vi "Begin.vi"(8 "error in":errorcluster) -> (0 "error out":errorcluster)   [LabVIEW 2015]
doc: "Called before other user functions, this VI is expected to open initial I/O refnums, load in file data, and do all program initialization. Notice that the <B>error out</B> terminal is simply used for data flow. Wiring it to other structures or subVIs ensures that this VI runs first."
uses:
  <vilib>/Rock Robotics/WPI/DriverStation/WPI_DriverStationRobotMode2.ctl
  <vilib>/Rock Robotics/WPI/Joystick/WPI_JoystickDeviceEnum.ctl
  <vilib>/Rock Robotics/WPI/Solenoid/WPI_SolenoidChannel.ctl
  <vilib>/Rock Robotics/SystemInterfaces/DIO/FPGA_DIOPWMChannel.ctl
  <vilib>/Rock Robotics/WPI/SafetyOutput/WPI_SafetyOutputConfigMenu.ctl
  Robot Global Data.vi
  <vilib>/Rock Robotics/Network Tables/NT Write String Array.vi
  <vilib>/Rock Robotics/WPI/Solenoid/WPI_SolenoidOpenSingle.vi
  <vilib>/Rock Robotics/WPI/MotorControl/WPI_MotorControlOpen Talon.vi
  <vilib>/Rock Robotics/WPI/MotorControl/WPI_MotorControlOpenCANTalonSRX.vi
  <vilib>/Rock Robotics/WPI/RobotDrive/WPI_RobotDriveOpen4MotorWithCANTalonSRX.vi
  <vilib>/Rock Robotics/WPI/Counter/WPI_CounterDigitalInputToDigitalSource.vi
  <vilib>/Rock Robotics/SystemInterfaces/DIO/FPGA_DIOChannel.ctl
  <vilib>/Rock Robotics/WPI/MotorControl/WPI_MotorControlOpen Victor.vi
  <vilib>/Rock Robotics/WPI/Gyro/WPI_GyroAnalogOpen.vi
  <vilib>/Rock Robotics/SystemInterfaces/AI/FPGA_AIGyroChannel.ctl
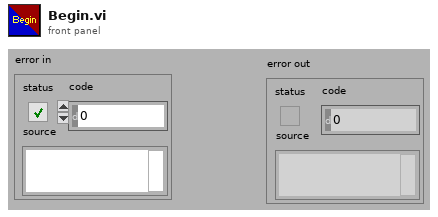
[diagram p1: front panel]
types:
  T1 = typedef "WPI_SafetyOutputConfigMenu.ctl" = enum16{"Enable", "Disable"}
  T2 = typedef "WPI_SolenoidChannel.ctl" = enum8{"Solenoid 0", "Solenoid 1", "Solenoid 2", "Solenoid 3", "Solenoid 4", "Solenoid 5", "Solenoid 6", "Solenoid 7", "Invalid"}
  T3 = typedef "FPGA_DIOPWMChannel.ctl" = enum8{"PWM 0", "PWM 1", "PWM 2", "PWM 3", "PWM 4", "PWM 5", "PWM 6", "PWM 7", "PWM 8", "PWM 9", "PWM MXP 0", "PWM MXP 1", "PWM MXP 2", "PWM MXP 3", "PWM MXP 4", "PWM MXP 5", "PWM MXP 6", "PWM MXP 7", "PWM MXP 8", "PWM MXP 9", "Invalid"}
  T4 = typedef "WPI_JoystickDeviceEnum.ctl" = enum16{"USB 0", "USB 1", "USB 2", "USB 3", "USB 4", "USB 5"}
  T5 = typedef "WPI_DriverStationRobotMode2.ctl" = enum16{"Autonomous Disabled", "Autonomous Enabled", "Teleop Disabled", "Teleop Enabled", "Disconnected", "Finish", "Test Disabled", "Test Enabled", "Emergency Stopped"}
  T6 = typedef "FPGA_DIOChannel.ctl" = enum8{"DIO 0", "DIO 1", "DIO 2", "DIO 3", "DIO 4", "DIO 5", "DIO 6", "DIO 7", "DIO 8", "DIO 9", "DIO MXP 0", "DIO MXP 1", "DIO MXP 2", "DIO MXP 3", "DIO MXP 4", "DIO MXP 5", "DIO MXP 6", "DIO MXP 7", "DIO MXP 8", "DIO MXP 9", "DIO MXP 10", "DIO MXP 11", "DIO MXP 12", "DIO MXP 13", "DIO MXP 14", "DIO MXP 15", "Invalid"}
  T7 = typedef "WPI_DigitalInputDevRef.ctl" = cluster{"DevStatus":errorcluster, "DIO Channel":T6}
  T8 = typedef "FPGA_CounterEncoderSourceConvertionLVSourceType.ctl" = cluster{"DevStatus":errorcluster, "AnalogTriggerMode?":bool, "DigitalMode":cluster{"DIO Channel":T9}, "AnalogTriggerMode":cluster{"AnalogTriggerIndex":T10, "OutputType":T11}}
  T9 = typedef "FPGA_DIODigitalSourceChannel.ctl" = enum8{"DIO 0", "DIO 1", "DIO 2", "DIO 3", "DIO 4", "DIO 5", "DIO 6", "DIO 7", "DIO 8", "DIO 9", "DIO MXP 0", "DIO MXP 1", "DIO MXP 2", "DIO MXP 3", "DIO MXP 4", "DIO MXP 5", "DIO MXP 6", "DIO MXP 7", "DIO MXP 8", "DIO MXP 9", "DIO MXP 10", "DIO MXP 11", "DIO MXP 12", "DIO MXP 13", "DIO MXP 14", "DIO MXP 15", "Disabled"}
  T10 = typedef "FPGA_AnalogTriggerIndex.ctl" = enum8{"Trig 0", "Trig 1", "Trig 2", "Trig 3", "Trig 4", "Trig 5", "Trig 6", "Trig 7", "Invalid"}
  T11 = typedef "FPGA_AnalogTriggerOutType.ctl" = enum16{"InWindow", "TriggerState", "Rising", "Falling"}
  T12 = typedef "WPI_EncoderDevRef.ctl" = cluster{"DevStatus":errorcluster, "EncoderIndex":T13, "CounterIndex":T14, "DistancePerCount":dbl, "Decoding Type":T15}
  T13 = typedef "FPGA_EncoderIdx.ctl" = enum8{"Enc 0", "Enc 1", "Enc 2", "Enc 3", "Enc 4", "Enc 5", "Enc 6", "Enc 7", "Invalid"}
  T14 = typedef "FPGA_CounterCtrSystemIndex.ctl" = enum8{"Ctr 0", "Ctr 1", "Ctr 2", "Ctr 3", "Ctr 4", "Ctr 5", "Ctr 6", "Ctr 7", "Invalid"}
  T15 = typedef "WPI_EncoderType.ctl" = enum16{"1x", "2x", "4x"}
  T16 = typedef "WPI_JoystickDevRef.ctl" = cluster{"Device":T4}
  T17 = typedef "WPI_SolenoidDevRef.ctl" = cluster{"DevStatus":errorcluster, "Pneumatics Control Module":u8, "Forward Solenoid Channel":T2, "Reverse Solenoid Channel":T2}
  T18 = typedef "WPI_MotorControlDeviceRef.ctl" = cluster{"DeviceStatus":errorcluster, "Type":T19, "PWM":cluster{"PWM Channel":T3, "DeadBand":T20}, "CAN":cluster{"Device Number":u8, "Control Mode":T21, "Semaphore":T22, "Max Vout":dbl, "TalonSRX Control Mode":T23}, "Invert":bool}
  T19 = typedef "WPI_MotorControlType.ctl" = enum16{"PWM", "CAN", "CANTalonSRX"}
  T20 = typedef "WPI_PWMDeadband.ctl" = cluster{"Name":string, "maxPositivePwm":i32, "minPositivePwm":i32, "centerPwm":i32, "maxNegativePwm":i32, "minNegativePwm":i32, "angularRange":u16}
  T21 = typedef "WPI_CANJaguar_ControlMode.ctl" = enum8{"Percent VBus", "Current", "Speed", "Position", "Voltage"}
  T22 = typedef "Semaphore RefNum" = refnum<k1>
  T23 = typedef "WPI_CANTalonSRX_APIControlMode.ctl" = enum8{"Percent VBus", "Speed", "Position", "Slave", "Unchanged / Invalid", "Voltage Compensation", "Current", "Motion Profile"}
  T24 = typedef "FPGA_AIGyroChannel.ctl" = enum8{"AI 0", "AI 1", "Invalid"}
  T25 = typedef "WPI_GyroDevRef.ctl" = cluster{"DevStatus":errorcluster, "Analog Channel":T26, "Offset":dbl, "Gain (VoltsPerDegree/Second)":dbl, "Gyro Type":enum16{"Analog", "XRS450"}, "Handle":i32, "SPI Bus":T27, "Device Found":bool, "Sample Rate":dbl, "Calibrate On Open":bool}
  T26 = typedef "FPGA_AIChannel.ctl" = enum8{"AI 0", "AI 1", "AI 2", "AI 3", "AI MXP 0", "AI MXP 1", "AI MXP 2", "AI MXP 3", "Invalid"}
  T27 = typedef "spi_bus.ctl" = enum16{"SPI On-Board, CS0", "SPI On-Board, CS1", "SPI On-Board, CS2", "SPI On-Board, CS3", "SPI MXP", "Invalid"}
  T28 = typedef "WPI_RobotDriveDevRef.ctl" = cluster{"DevStatus":errorcluster, "Motors[]":T18[], "Square Inputs":bool, "Max Output":dbl}
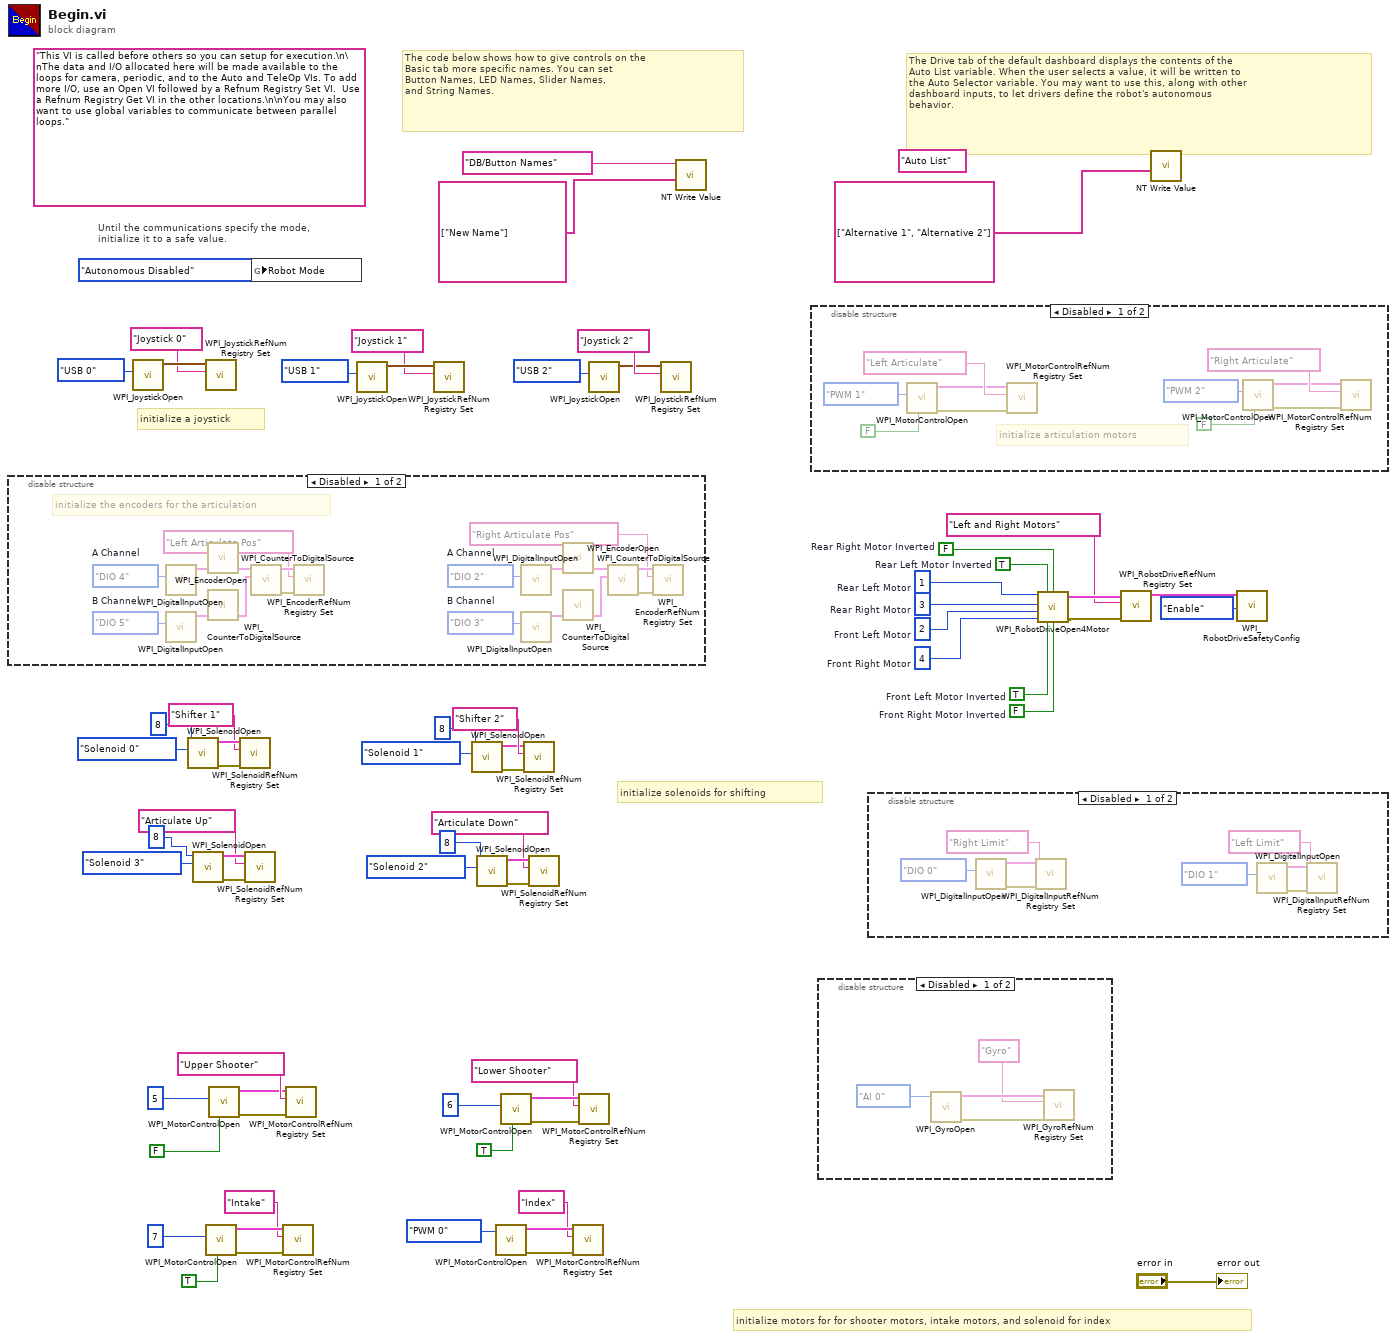
[diagram p0: block diagram]
diagram:
  w13 = u8 4  # Front Right Motor
  w12 = u8 3  # Rear Right Motor
  w11 = u8 2  # Front Left Motor
  w10 = u8 1  # Rear Left Motor
  w9 = TRUE  # Rear Left Motor Inverted
  w8 = FALSE  # Rear Right Motor Inverted
  w7 = FALSE  # Front Right Motor Inverted
  w6 = TRUE  # Front Left Motor Inverted
  (unwired) "This VI is called before others so you can setup for execution.\n\nThe data and I/O allocated here will be made available to the loops for camera, periodic, and to the Auto and TeleOp VIs. To add more I/O, use an Open VI followed by a Refnum Registry Set VI.  Use a Refnum Registry Get VI in the other locations.\n\nYou may also want to use global variables to communicate between parallel loops."
  # "initialize solenoids for shifting"
  # "initialize a joystick"
  # "initialize motors for for shooter motors, intake motors, and solenoid for index"
  # "The Drive tab of the default dashboard displays the contents of the\nAuto List variable. When the user selects a value, it will be written to\nthe Auto Selector variable. You may want to use this, along with other\ndashboard inputs, to let drivers define the robot's autonomous\nbehavior."
  # "The code below shows how to give controls on the\nBasic tab more specific names. You can set\nButton Names, LED Names, Slider Names,\nand String Names."
  # "Until the communications specify the mode,\ninitialize it to a safe value."
  n1 = disable-structure shown="Disabled" {
    frame Disabled {
      w69 = FPGA_DIOChannel."DIO 5"  # B Channel
      w70 = FPGA_DIOChannel."DIO 4"  # A Channel
      w85 = FPGA_DIOChannel."DIO 3"  # B Channel
      w84 = FPGA_DIOChannel."DIO 2"  # A Channel
      # "initialize the encoders for the articulation"
      n2 = call <vilib>:"WPI_DigitalInputOpen.vi"("DIO Channel"=w70) -> ("DigitalInputDevRef"=w73:T7)  [unwired: 1 in, 9 out]
      n3 = call <vilib>:"WPI_DigitalInputOpen.vi"("DIO Channel"=w69) -> ("DigitalInputDevRef"=w72:T7)  [unwired: 1 in, 9 out]
      n4 = call-poly <vilib>:"WPI_CounterToDigitalSource.vi"("DigitalInputDevRef"=w73) -> ("Digital Source"=w74:T8)  [unwired: 6 out]
      n5 = call-poly <vilib>:"WPI_CounterToDigitalSource.vi"("DigitalInputDevRef"=w72) -> ("Digital Source"=w71:T8)  [unwired: 6 out]
      n6 = call <vilib>:"WPI_EncoderOpen.vi"("BSource"=w71, "ASource"=w74) -> ("error out"=w75:errorcluster, "EncoderDevRef"=w76:T12)  [unwired: 6 in, 2 out]
      n7 = call <vilib>:"WPI_EncoderRefNum Registry Set.vi"("error in (no error)"=w75, "refnum name"="Left Articulate Pos", "EncoderDevRef"=w76) -> ()  [unwired: 7 in, 2 out]
      n8 = call <vilib>:"WPI_DigitalInputOpen.vi"("DIO Channel"=w84) -> ("DigitalInputDevRef"=w81:T7)  [unwired: 1 in, 9 out]
      n9 = call <vilib>:"WPI_DigitalInputOpen.vi"("DIO Channel"=w85) -> ("DigitalInputDevRef"=w82:T7)  [unwired: 1 in, 9 out]
      n10 = call-poly <vilib>:"WPI_CounterToDigitalSource.vi"("DigitalInputDevRef"=w81) -> ("Digital Source"=w80:T8)  [unwired: 6 out]
      n11 = call-poly <vilib>:"WPI_CounterToDigitalSource.vi"("DigitalInputDevRef"=w82) -> ("Digital Source"=w83:T8)  [unwired: 6 out]
      n12 = call <vilib>:"WPI_EncoderOpen.vi"("BSource"=w83, "ASource"=w80) -> ("error out"=w79:errorcluster, "EncoderDevRef"=w78:T12)  [unwired: 6 in, 2 out]
      n13 = call <vilib>:"WPI_EncoderRefNum Registry Set.vi"("error in (no error)"=w79, "refnum name"="Right Articulate Pos", "EncoderDevRef"=w78) -> ()  [unwired: 7 in, 2 out]
    }
    frame Enabled {
    }
  }
  n14 = call <vilib>:"WPI_JoystickOpen.vi"("JoystickDevice"=WPI_JoystickDeviceEnum."USB 0") -> ("JoystickDevRef"=w60:T16)  [unwired: 10 in]
  n15 = call-poly <vilib>:"WPI_SolenoidOpen.vi"("Solenoid Channel"=WPI_SolenoidChannel."Solenoid 0", "Pneumatics Control Module (0)"=u8 8) -> ("error out"=w52:errorcluster, "SolenoidDevRef"=w51:T17)  [unwired: 8 in]
  n16 = call-poly <vilib>:"WPI_SolenoidOpen.vi"("Solenoid Channel"=WPI_SolenoidChannel."Solenoid 3", "Pneumatics Control Module (0)"=u8 8) -> ("error out"=w32:errorcluster, "SolenoidDevRef"=w33:T17)  [unwired: 8 in]
  n17 = call <vilib>:"WPI_JoystickRefNum Registry Set.vi"("refnum name"="Joystick 0", "JoystickDevRef"=w60) -> ()  [unwired: 8 in, 2 out]
  n18 = call-poly <vilib>:"WPI_MotorControlOpen.vi"("Invert"=TRUE, "Device Number"=u8 7) -> ("error out"=w18:errorcluster, "MotorControlDeviceRef"=w17:T18)  [unwired: 8 in]
  n19 = call-poly <vilib>:"WPI_MotorControlOpen.vi"("Invert"=FALSE, "Device Number"=u8 5) -> ("error out"=w26:errorcluster, "MotorControlDeviceRef"=w27:T18)  [unwired: 8 in]
  n20 = call <vilib>:"WPI_SolenoidRefNum Registry Set.vi"("error in (no error)"=w52, "refnum name"="Shifter 1", "SolenoidDevRef"=w51) -> ()  [unwired: 7 in, 2 out]
  n21 = call <vilib>:"WPI_SolenoidRefNum Registry Set.vi"("error in (no error)"=w32, "refnum name"="Articulate Up", "SolenoidDevRef"=w33) -> ()  [unwired: 7 in, 2 out]
  n22 = global write "Robot Global Data.vi" "Robot Mode"(WPI_DriverStationRobotMode2."Autonomous Disabled" ("Robot Mode")) -> ()
  n23 = call <vilib>:"WPI_MotorControlRefNum Registry Set.vi"("error in (no error)"=w18, "refnum name"="Intake", "MotorControlDevRef"=w17) -> ()  [unwired: 7 in, 2 out]
  n24 = call <vilib>:"WPI_MotorControlRefNum Registry Set.vi"("error in (no error)"=w26, "refnum name"="Upper Shooter", "MotorControlDevRef"=w27) -> ()  [unwired: 7 in, 2 out]
  n25 = call <vilib>:"WPI_JoystickOpen.vi"("JoystickDevice"=WPI_JoystickDeviceEnum."USB 1") -> ("JoystickDevRef"=w57:T16)  [unwired: 10 in]
  n26 = call <vilib>:"WPI_JoystickRefNum Registry Set.vi"("refnum name"="Joystick 1", "JoystickDevRef"=w57) -> ()  [unwired: 8 in, 2 out]
  n27 = call-poly <vilib>:"WPI_SolenoidOpen.vi"("Solenoid Channel"=WPI_SolenoidChannel."Solenoid 1", "Pneumatics Control Module (0)"=u8 8) -> ("error out"=w45:errorcluster, "SolenoidDevRef"=w46:T17)  [unwired: 8 in]
  n28 = call-poly <vilib>:"WPI_SolenoidOpen.vi"("Solenoid Channel"=WPI_SolenoidChannel."Solenoid 2", "Pneumatics Control Module (0)"=u8 8) -> ("error out"=w37:errorcluster, "SolenoidDevRef"=w36:T17)  [unwired: 8 in]
  n29 = call-poly <vilib>:"WPI_MotorControlOpen.vi"("PWM Channel"=FPGA_DIOPWMChannel."PWM 0") -> ("error out"=w42:errorcluster, "MotorControlDeviceRef"=w41:T18)  [unwired: 9 in]
  n30 = call-poly <vilib>:"WPI_MotorControlOpen.vi"("Invert"=TRUE, "Device Number"=u8 6) -> ("error out"=w25:errorcluster, "MotorControlDeviceRef"=w24:T18)  [unwired: 8 in]
  n31 = call <vilib>:"WPI_SolenoidRefNum Registry Set.vi"("error in (no error)"=w45, "refnum name"="Shifter 2", "SolenoidDevRef"=w46) -> ()  [unwired: 7 in, 2 out]
  n32 = call <vilib>:"WPI_SolenoidRefNum Registry Set.vi"("error in (no error)"=w37, "refnum name"="Articulate Down", "SolenoidDevRef"=w36) -> ()  [unwired: 7 in, 2 out]
  n33 = call <vilib>:"WPI_MotorControlRefNum Registry Set.vi"("error in (no error)"=w42, "refnum name"="Index", "MotorControlDevRef"=w41) -> ()  [unwired: 7 in, 2 out]
  n34 = call <vilib>:"WPI_MotorControlRefNum Registry Set.vi"("error in (no error)"=w25, "refnum name"="Lower Shooter", "MotorControlDevRef"=w24) -> ()  [unwired: 7 in, 2 out]
  n35 = call <vilib>:"WPI_JoystickOpen.vi"("JoystickDevice"=WPI_JoystickDeviceEnum."USB 2") -> ("JoystickDevRef"=w54:T16)  [unwired: 10 in]
  n36 = call <vilib>:"WPI_JoystickRefNum Registry Set.vi"("refnum name"="Joystick 2", "JoystickDevRef"=w54) -> ()  [unwired: 8 in, 2 out]
  n37 = call-poly <vilib>:"NT Write Value.vi"("String Array"=string[] ["New Name"], "Name"="DB/Button Names") -> ()  [unwired: 9 in, 1 out]
  n38 = disable-structure shown="Disabled" {
    frame Disabled {
      # "initialize articulation motors"
      n39 = call-poly <vilib>:"WPI_MotorControlOpen.vi"("Invert"=FALSE ("Invert Left"), "PWM Channel"=FPGA_DIOPWMChannel."PWM 1") -> ("error out"=w91:errorcluster, "MotorControlDeviceRef"=w92:T18)  [unwired: 8 in]
      n40 = call <vilib>:"WPI_MotorControlRefNum Registry Set.vi"("error in (no error)"=w91, "refnum name"="Left Articulate", "MotorControlDevRef"=w92) -> ()  [unwired: 7 in, 2 out]
      n41 = call-poly <vilib>:"WPI_MotorControlOpen.vi"("Invert"=FALSE ("Invert Right"), "PWM Channel"=FPGA_DIOPWMChannel."PWM 2") -> ("error out"=w88:errorcluster, "MotorControlDeviceRef"=w89:T18)  [unwired: 8 in]
      n42 = call <vilib>:"WPI_MotorControlRefNum Registry Set.vi"("error in (no error)"=w88, "refnum name"="Right Articulate", "MotorControlDevRef"=w89) -> ()  [unwired: 7 in, 2 out]
    }
    frame Enabled {
    }
  }
  n43 = disable-structure shown="Disabled" {
    frame Disabled {
      n44 = call-poly <vilib>:"WPI_GyroOpen.vi"("Analog Channel"=FPGA_AIGyroChannel."AI 0") -> ("error out"=w98:errorcluster, "GyroDevRef"=w99:T25)  [unwired: 8 in, 1 out]
      n45 = call <vilib>:"WPI_GyroRefNum Registry Set.vi"("error in (no error)"=w98, "refnum name"="Gyro", "GyroDevRef"=w99) -> ()  [unwired: 7 in, 2 out]
    }
    frame Enabled {
    }
  }
  n46 = disable-structure shown="Disabled" {
    frame Disabled {
      n47 = call <vilib>:"WPI_DigitalInputOpen.vi"("DIO Channel"=FPGA_DIOChannel."DIO 0") -> ("error out"=w106:errorcluster, "DigitalInputDevRef"=w105:T7)  [unwired: 9 in]
      n48 = call <vilib>:"WPI_DigitalInputRefNum Registry Set.vi"("error in (no error)"=w106, "refnum name"="Right Limit", "DigitalInputDevRef"=w105) -> ()  [unwired: 7 in, 2 out]
      n49 = call <vilib>:"WPI_DigitalInputOpen.vi"("DIO Channel"=FPGA_DIOChannel."DIO 1") -> ("error out"=w103:errorcluster, "DigitalInputDevRef"=w104:T7)  [unwired: 9 in]
      n50 = call <vilib>:"WPI_DigitalInputRefNum Registry Set.vi"("error in (no error)"=w103, "refnum name"="Left Limit", "DigitalInputDevRef"=w104) -> ()  [unwired: 7 in, 2 out]
    }
    frame Enabled {
    }
  }
  n51 = call-poly <vilib>:"WPI_RobotDriveOpen4Motor.vi"("Rear Left Motor"=w10, "Rear Left Motor Inverted"=w9, "Rear Right Motor Inverted"=w8, "Rear Right Motor"=w12, "Front Left Motor"=w11, "Front Right Motor"=w13, "Front Left Motor Inverted"=w6, "Front Right Motor Inverted"=w7) -> ("RobotDriveDevRef"=w4:T28, "error out"=w5:errorcluster)  [unwired: 6 in]
  n52 = call <vilib>:"WPI_RobotDriveRefNum Registry Set.vi"("error in (no error)"=w5, "refnum name"="Left and Right Motors", "RobotDriveDevRef"=w4) -> ("RobotDriveDevRef"=w2:T28)  [unwired: 1 in, 7 out]
  n53 = call-poly <vilib>:"NT Write Value.vi"("String Array"=string[] ["Alternative 1", "Alternative 2"], "Name"="Auto List") -> ()  [unwired: 9 in, 1 out]
  n54 = call <vilib>:"WPI_RobotDriveSafetyConfig.vi"("mode"=WPI_SafetyOutputConfigMenu."Enable", "RobotDriveDevRef"=w2) -> ()  [unwired: 8 in, 2 out]
  "error out" <- "error in"
